vi "swerve_math.vi"(0 "Strafe":dbl(slide) scale=-1.0..1.0, 2 "Forwards":dbl(slide) scale=-1.0..1.0, 4 "Rotate":dbl(slide) scale=-1.0..1.0, 6 "Gyro":dbl) -> (20 "Drive FR":dbl, 21 "Azimuth FR":dbl, 22 "Drive FL":dbl, 23 "Azimuth FL":dbl, 24 "Drive BL":dbl, 25 "Azimuth BL":dbl, 26 "Drive BR":dbl, 27 "Azimuth BR":dbl)   [LabVIEW 2020]
uses:
  <vilib>/Analysis/coordinate.llb/Angle Units.ctl
  <vilib>/Analysis/coordinate.llb/Wrap Angle (scalar).vi
  <vilib>/Analysis/coordinate.llb/2D Cartesian Coordinate Rotation (Scalar).vi
  <vilib>/Analysis/NI_AALPro.lvlib
  <vilib>/Analysis/NI_AAL_Angle.lvlib
panel:
  out "Back Right":cluster{"X":dbl, "Y":dbl}[](graph)
  out "Back Left":cluster{"X":dbl, "Y":dbl}[](graph)
  out "Front Right":cluster{"X":dbl, "Y":dbl}[](graph)
  out "Front Left":cluster{"X":dbl, "Y":dbl}[](graph)
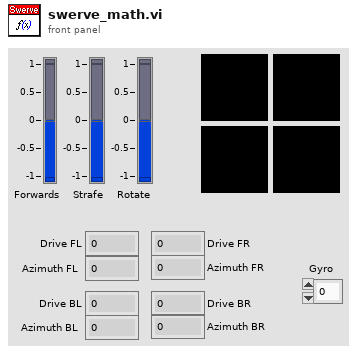
[diagram p1: front panel]
types:
  T1 = typedef "NI_AAL_Angle.lvlib/Angle Units.ctl" = i32
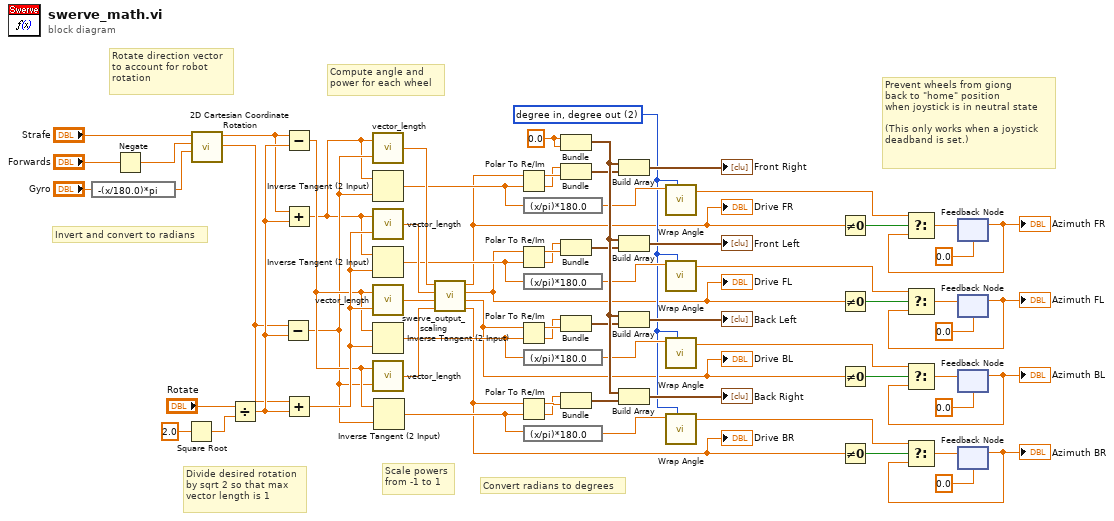
[diagram p0: block diagram]
diagram:
  w26 = T1 2 items=["radian in, radian out", "radian in, degree out", "degree in, degree out", "degree in, radian out"] ("angle units")
  w66 = 0.0 ("x")
  # "Prevent wheels from giong\nback to \"home\" position\nwhen joystick is in neutral state\n\n(This only works when a joystick\ndeadband is set.)"
  # "Divide desired rotation\nby sqrt 2 so that max\nvector length is 1"
  # "Convert radians to degrees"
  # "Scale powers\nfrom -1 to 1"
  # "Compute angle and \npower for each wheel"
  # "Rotate direction vector\nto account for robot \nrotation"
  # "Invert and convert to radians"
  n1 = expression code="-(x/180.0)*pi" ("degrees to radians")("Gyro") -> (w31:dbl)
  n2 = Negate(x="Forwards") -> (-x=w25:dbl)
  n3 = Square Root(x=2.0) -> (sqrt(x)=w70:dbl)
  n4 = call-poly <vilib>:"2D Cartesian Coordinate Rotation.vi"("theta"=w31, "y"=w25, "x"="Strafe") -> ("y out"=w33:dbl, "x out"=w34:dbl)  [unwired: 6 in, 1 out]
  n5 = Divide(x="Rotate", y=w70) -> (x/y=w67:dbl)
  n6 = Subtract(x=w33, y=w67) -> (x-y=w46:dbl)
  n7 = Subtract(x=w34, y=w67) -> (x-y=w47:dbl)
  n8 = Add(x=w34, y=w67) -> (x+y=w45:dbl)
  n9 = Add(x=w33, y=w67) -> (x+y=w48:dbl)
  n10 = call "vector_length.vi"("v_y"=w46, "v_x"=w45) -> ("||v||"=w56:dbl)
  n11 = Inverse Tangent (2 Input)(1:w46, 2:w45) -> (0:w49:dbl)
  n12 = call "vector_length.vi"("v_y"=w48, "v_x"=w45) -> ("||v||"=w55:dbl)
  n13 = Inverse Tangent (2 Input)(1:w48, 2:w45) -> (0:w50:dbl)
  n14 = call "vector_length.vi"("v_y"=w48, "v_x"=w47) -> ("||v||"=w54:dbl)
  n15 = Inverse Tangent (2 Input)(1:w48, 2:w47) -> (0:w51:dbl)
  n16 = call "vector_length.vi"("v_y"=w46, "v_x"=w47) -> ("||v||"=w53:dbl)
  n17 = Inverse Tangent (2 Input)(1:w46, 2:w47) -> (0:w52:dbl)
  n18 = call "swerve_output_scaling.vi"("d"=w53, "c"=w54, "b"=w55, "a"=w56) -> ("d scaled"=w4:dbl, "c scaled"=w3:dbl, "b scaled"=w2:dbl, "a scaled"=w1:dbl)  [unwired: 4 in]
  "Drive FR" <- w1
  "Drive FL" <- w2
  "Drive BL" <- w3
  "Drive BR" <- w4
  n19 = Polar To Re/Im(2:w49, 3:w1) -> (0:w43:dbl, 1:w44:dbl)
  n20 = Polar To Re/Im(2:w50, 3:w2) -> (0:w41:dbl, 1:w42:dbl)
  n21 = Polar To Re/Im(2:w51, 3:w3) -> (0:w39:dbl, 1:w40:dbl)
  n22 = Polar To Re/Im(2:w52, 3:w4) -> (0:w37:dbl, 1:w38:dbl)
  n23 = expression code="(x/pi)*180.0" ("radians to degrees")(w49) -> (w30:dbl)
  n24 = expression code="(x/pi)*180.0" ("radians to degrees")(w50) -> (w29:dbl)
  n25 = expression code="(x/pi)*180.0" ("radians to degrees")(w51) -> (w28:dbl)
  n26 = expression code="(x/pi)*180.0" ("radians to degrees")(w52) -> (w27:dbl)
  n27 = Bundle("x"=w66, "x"=w66) -> (w65:cluster{"x":dbl, "x":dbl})  [unwired: 1 in]
  n28 = Bundle(w43, w44) -> (w59:cluster{dbl, dbl})  [unwired: 1 in]
  n29 = Bundle(w41, w42) -> (w60:cluster{dbl, dbl})  [unwired: 1 in]
  n30 = Bundle(w39, w40) -> (w58:cluster{dbl, dbl})  [unwired: 1 in]
  n31 = Bundle(w37, w38) -> (w57:cluster{dbl, dbl})  [unwired: 1 in]
  n32 = Build Array(w65, w59) -> (→"Front Right":cluster{"x":dbl, "x":dbl}[])
  n33 = Build Array(w65, w60) -> (→"Front Left":cluster{"x":dbl, "x":dbl}[])
  n34 = Build Array(w65, w58) -> (→"Back Left":cluster{"x":dbl, "x":dbl}[])
  n35 = Build Array(w65, w57) -> (→"Back Right":cluster{"x":dbl, "x":dbl}[])
  n36 = call-poly <vilib>:"Wrap Angle.vi"("angle units"=w26, "angle in"=w30) -> ("angle out"=w23:dbl)  [unwired: 8 in, 1 out]
  n37 = call-poly <vilib>:"Wrap Angle.vi"("angle units"=w26, "angle in"=w29) -> ("angle out"=w14:dbl)  [unwired: 8 in, 1 out]
  n38 = call-poly <vilib>:"Wrap Angle.vi"("angle units"=w26, "angle in"=w28) -> ("angle out"=w13:dbl)  [unwired: 8 in, 1 out]
  n39 = call-poly <vilib>:"Wrap Angle.vi"("angle units"=w26, "angle in"=w27) -> ("angle out"=w12:dbl)  [unwired: 8 in, 1 out]
  n40 = Not Equal To 0?(x=w1) -> (x != 0?=w24:bool)
  n41 = Not Equal To 0?(x=w2) -> (x != 0?=w15:bool)
  n42 = Not Equal To 0?(x=w3) -> (x != 0?=w18:bool)
  n43 = Not Equal To 0?(x=w4) -> (x != 0?=w16:bool)
  n44 = feedback #1(0.0 ("angle out")) -> (w11:dbl)
  "Azimuth FR" <- w11
  n45 = Select(t=w23, s=w24, f=w11) -> (s? t:f=w22:dbl)
  n46 = feedback-in #1(w22) -> ()
  n47 = feedback #2(0.0 ("angle out")) -> (w10:dbl)
  "Azimuth FL" <- w10
  n48 = Select(t=w14, s=w15, f=w10) -> (s? t:f=w20:dbl)
  n49 = feedback-in #2(w20) -> ()
  n50 = feedback #3(0.0 ("angle out")) -> (w9:dbl)
  "Azimuth BL" <- w9
  n51 = Select(t=w13, s=w18, f=w9) -> (s? t:f=w19:dbl)
  n52 = feedback-in #3(w19) -> ()
  n53 = feedback #4(0.0 ("angle out")) -> (w8:dbl)
  "Azimuth BR" <- w8
  n54 = Select(t=w12, s=w16, f=w8) -> (s? t:f=w17:dbl)
  n55 = feedback-in #4(w17) -> ()
